vi "dfd_Validate MRate NStage FXP for Code Gen.vi"(7 "totalChan":i32=3, 8 "error in":errorcluster, 11 "multirate filters":T1[](array[typedef]) {"mMRate_SumWl" min=1 max=32 step=1; "mMRate_InputIwl" min=1 max=32 step=1; "mMRate_GainWl" min=1 max=32 step=1; "mMRate_OutputWl" min=1 max=32 step=1; "mMRate_InputWl" min=1 max=32 step=1; "mMRate_CoefWl" min=1 max=32 step=1; "mMRate_Mode" items=["Default"=-1, "No Rate Change"=0, "Interpolation"=1, "Decimation"=2, "Interpolated"=3, "Rational"=4]}) -> (0 "error out":errorcluster, 3 "multirate filters out":T1[](array[typedef]) {"mMRate_SumWl" min=1 max=32 step=1; "mMRate_InputIwl" min=1 max=32 step=1; "mMRate_GainWl" min=1 max=32 step=1; "mMRate_OutputWl" min=1 max=32 step=1; "mMRate_InputWl" min=1 max=32 step=1; "mMRate_CoefWl" min=1 max=32 step=1; "mMRate_Mode" items=["Default"=-1, "No Rate Change"=0, "Interpolation"=1, "Decimation"=2, "Interpolated"=3, "Rational"=4]})   [LabVIEW 2017, in "NI_DigFilterLicensed.lvlib"]
uses:
  <vilib>/addons/Digital Filter Design/NI_DigFilterLicensed.lvlib
  <vilib>/addons/Digital Filter Design/_Objects.llb/DFD Multirate Filter Obj.ctl
  <vilib>/addons/Digital Filter Design/_Objects.llb/DFD Multirate Mode.ctl
  <vilib>/addons/Digital Filter Design/_Objects.llb/DFD Coef Norm Type.ctl
  <vilib>/addons/Digital Filter Design/_Objects.llb/DFD Round-off Mode.ctl
  <vilib>/addons/Digital Filter Design/_Objects.llb/DFD FXP MRate Multiply Mode.ctl
  <vilib>/addons/Digital Filter Design/_Misc.llb/dfd_Error Handlers (Single).vi
  <vilib>/addons/Digital Filter Design/NI_DigFilter_FXP.lvlib
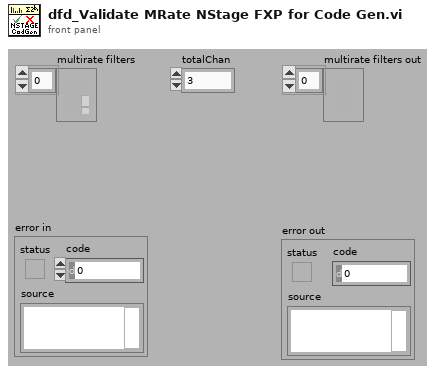
[diagram p1: front panel]
types:
  T1 = typedef "NI_DigFilterLicensed.lvlib/DFD Multirate Filter Obj.ctl" = cluster{"mMRate_Structure":enum16{"CIC", "FIR", "IIR", "Lattice"}, "mMRate_Mode":T2, "mMRate_Factor":i32, "mMRate_FIRParams":cluster{"mMRate_FIR_H":dbl[], "mMRate_FIR_IsNyquist?":bool, "mMRate_FIR_IsSymmetric?":bool}, "mMRate_CICParams":cluster{"mMRate_CIC_#Stage":i32, "mMRate_CIC_Lag":i32, "mMRate_CIC_Type":enum16{"Lowpass", "Highpass"}}, "mMRate_Order":i32, "mMRate_Version":string, "mMRate_Comments":string, "mMRate_RationalFactor":cluster{"mMRate_L":i32, "mMRate_M":i32}, "mMRate_Fs":dbl, "mMRate_Quantized?":bool, "mMRate_QFilterGain":dbl, "mMRate_CoefWl":i16, "mMRate_Scaling":cluster{"mMRate_ScaleByPowerOf2?":bool, "mMRate_ScaleType":T3}, "mMRate_InputWl":i16, "mMRate_OutputWl":i16, "mMRate_OutputMode":T4, "mMRate_MultMode":T5, "mMRate_BitPruning":bool, "mMRate_GainWl":i16, "mMRate_OutputFwl":i16, "mMRate_SumIwl":i16, "mMRate_InputIwl ":i16, "mMRate_SumWl":i16, "mMRate_CoefIwl":i16}
  T2 = typedef "NI_DigFilterLicensed.lvlib/DFD Multirate Mode.ctl" = i16
  T3 = typedef "NI_DigFilterLicensed.lvlib/DFD Coef Norm Type.ctl" = enum16{"No Norm", "Time Domain 1-Norm", "Time Domain 2-Norm", "Time Domain Inf-Norm"}
  T4 = typedef "NI_DigFilterLicensed.lvlib/DFD Round-off Mode.ctl" = enum16{"Nearest", "Truncation"}
  T5 = typedef "NI_DigFilterLicensed.lvlib/DFD FXP MRate Multiply Mode.ctl" = enum16{"Truncated", "Full"}
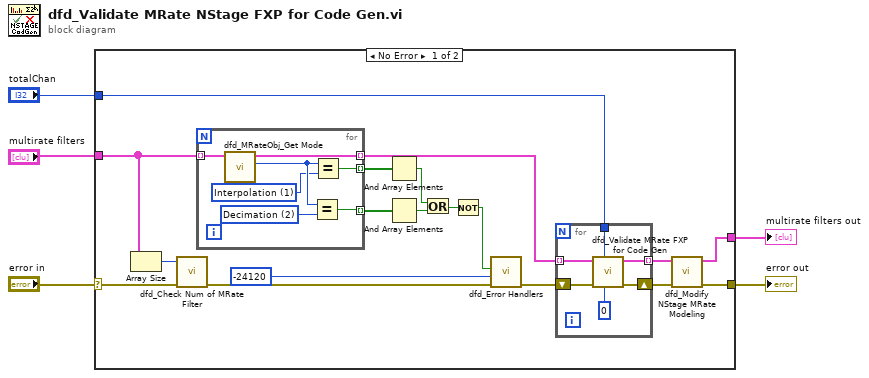
[diagram p0: block diagram]
diagram:
  n1 = case shown="No Error" "error in" {
    selector: "error in" -> [w6 w37]
    tunnel: [w21 _] -> w5
    tunnel: [w19 w37] -> w4
    tunnel: "totalChan" -> [w18 _]
    tunnel: "multirate filters" -> [w17 _]
    frame No Error {
      n2 = Array Size(array=w17) -> (size(s)=w23:i32)
      n3 = call <vilib>:"dfd_Check Num of MRate Filter.vi"("error in (no error)"=w6, "#MRate in"=w23) -> ("error out"=w9:errorcluster)  [unwired: 9 out]
      n4 = for {
        tunnel: w17 -> [w30] mode=indexing
        tunnel: [w29] -> w16 mode=indexing
        tunnel: [w25] -> w15 mode=indexing
        tunnel: [w24] -> w14 mode=indexing
        w28 = T2 2 items=["Default"=-1, "No Rate Change"=0, "Interpolation"=1, "Decimation"=2, "Interpolated"=3, "Rational"=4] ("y")
        w26 = T2 1 items=["Default"=-1, "No Rate Change"=0, "Interpolation"=1, "Decimation"=2, "Interpolated"=3, "Rational"=4] ("y")
        n5 = call <vilib>:"dfd_MRateObj_Get Mode.vi"("multirate filter in"=w30) -> ("mode"=w27:T2, "dup multirate filter"=w29:T1)  [unwired: 9 out]
        n6 = Equal?(x=w27, y=w28) -> (x = y?=w24:bool)
        n7 = Equal?(x=w27, y=w26) -> (x = y?=w25:bool)
      }
      n8 = And Array Elements(Boolean array=w15) -> (logical AND=w13:bool)
      n9 = And Array Elements(Boolean array=w14) -> (logical AND=w12:bool)
      n10 = Or(x=w13, y=w12) -> (x .or. y?=w11:bool)
      n11 = Not(x=w11) -> (.not. x?=w10:bool)
      n12 = call-poly <vilib>:"dfd_Error Handlers.vi"("error in (no error)"=w9, "error code"=-24120 ("ERR_MULTISTAGE_MULT_CODEGEN_MODE"), "condition failed?"=w10) -> ("error out"=w7:errorcluster)  [unwired: 8 out]
      n13 = for {
        tunnel: [w33] -> w22 mode=indexing
        tunnel: w16 -> [w36] mode=indexing
        shift-right: [w34] -> w20
        shift-left: w7 -> [w35]
        tunnel: w18 -> [w32]
        n14 = call <vilib>:"dfd_Validate MRate FXP for Code Gen.vi"("output phase"=0, "totalChan"=w32, "error in"=w35, "multirate filter"=w36) -> ("error out"=w34:errorcluster, "multirate filter out"=w33:T1)  [unwired: 6 out]
      }
      n15 = call <vilib>:"dfd_Modify NStage MRate Modeling.vi"("error in (no error)"=w20, "multirate filters in"=w22) -> ("error out"=w19:errorcluster, "multirate filters out"=w21:T1[])  [unwired: 8 out]
    }
    frame Error {
    }
  }
  "error out" <- w4
  "multirate filters out" <- w5
